vi "Write FIFO Header to CIPC.vi"(8 "error in (no error)":errorcluster, 9 "Payload Length (bytes)":i32, 10 "FIFO Timestamps":T1, 11 "CIF_CIPC_Chn in":refnum<class "CIF_CIPC_Chn.lvclass">) -> (0 "error out":errorcluster, 3 "CIF_CIPC_Chn out":refnum<class "CIF_CIPC_Chn.lvclass">)   [LabVIEW 2021, in "CIF_CIPC_Chn.lvclass"]
uses:
  CIF_CIPC_Chn.lvclass
  CIF_CIPC_Chn.lvclass/CIF_CIPC_Chn.ctl
  CIFChannels/CIFChannels.lvclass
  <vilib>/CIF Foundation/CIF CIPC/TypeDefs/Partial Write Configuration.ctl
  <vilib>/CIF Foundation/CIF CIPC/CIF_NI_CIPC.lvlib
  2516c5c4-bcd6-4eab-a054-fa3d4f1376bc.vi
  D:/dev/Packages/CIF_Channels_Core/src/CIFChannels/CIFChannels.lvclass
  D:/dev/Packages/CIF_Channels_Core/src/CIPC_Channels/CIF_CIPC_Chan/CIF_CIPC_Chn.lvclass
  ChannelCommon/typedef/TimeStamps.ctl
  ChannelCommon/ChannelCommon.lvlib
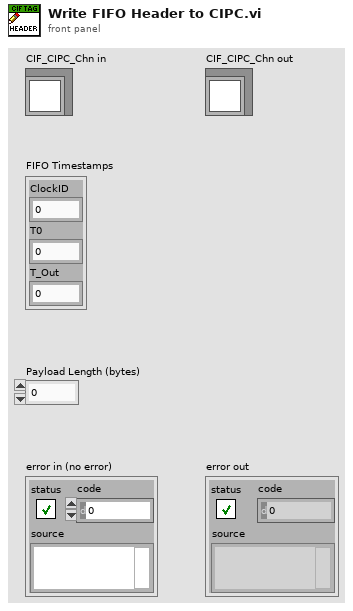
[diagram p1: front panel]
types:
  T1 = typedef "ChannelCommon.lvlib/TimeStamps.ctl" = cluster{"ClockID":u8, "T0":i64, "T_Out":i64}
  T2 = typedef "CIF_NI_CIPC.lvlib/Partial Write Configuration.ctl" = cluster{"Start Offset (bytes)":u32, "Total Length (bytes)":u32, "Last Write":bool, "Get Write Position":bool, "Notify Readers":bool}
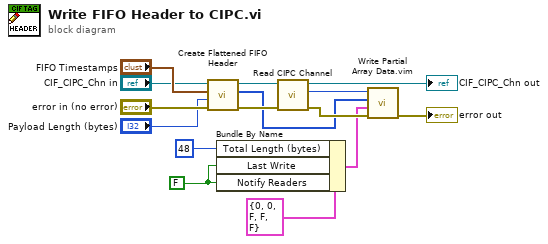
[diagram p0: block diagram]
diagram:
  w8 = FALSE ("Last Write")
  n1 = call "Create Flattened FIFO Header.vi"("error in (no error)"="error in (no error)", "Data Length"="Payload Length (bytes)", "FIFO Timestamps"="FIFO Timestamps", "CIFChannels in"="CIF_CIPC_Chn in") -> ("error out"=w4:errorcluster, "Flattened FIFO Header"=w3:u8[], "CIFChannels out"=w6:refnum<class "CIF_CIPC_Chn.lvclass">)  [unwired: 5 in]
  n2 = Bundle By Name(cluster=T2 {"Start Offset (bytes)"=0, "Total Length (bytes)"=0, "Last Write"=FALSE, "Get Write Position"=FALSE, "Notify Readers"=FALSE} ("Partial Write Configuration"), "Total Length (bytes)"=u32 48 ("y"), "Last Write"=w8, "Notify Readers"=w8) -> (w7:T2)
  n3 = call "Read CIPC Channel.vi"("error in (no error)"=w4, "CIFTag in"=w6) -> ("error out"=w10:errorcluster, "CIF Channel"=w11:u64, "CIFTag out"=→"CIF_CIPC_Chn out":refnum<class "CIF_CIPC_Chn.lvclass">)  [unwired: 7 in]
  n4 = call "Write Partial Array Data.vim"("error in (no error)"=w10, "Partial Write Configuration"=w7, "Data in"=w3, "CIPC Reference in"=w11) -> ("error out"=→"error out":errorcluster)  [unwired: 4 in, 3 out]
